vi "CLD 13 Flow Rates Exercise.vi"() -> ()   [LabVIEW 2009]
doc: "CLD 13 exercise"
panel:
  out "Error Out":errorcluster
  in  "Error In":errorcluster
  out "Flow Rate Meter":i8(knob) scale format="%_2f"
  in  "Stop Application":bool
  in  "Stop Flow":bool
  out "Elapsed Time":dbl
  out "Flow Rate":dbl
  in  "Flow Rate Change":i8(slide) min=-2 max=2 step=1
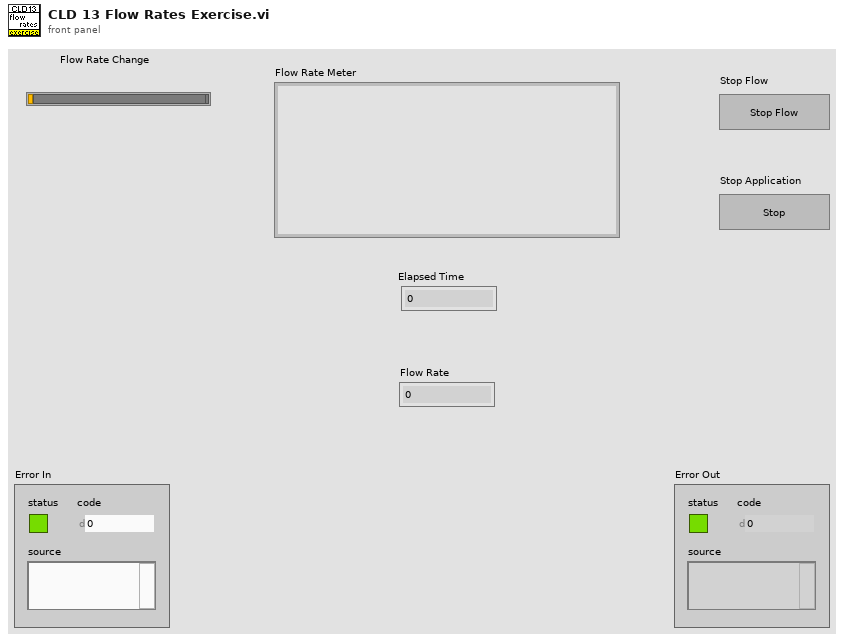
[diagram p1: front panel]
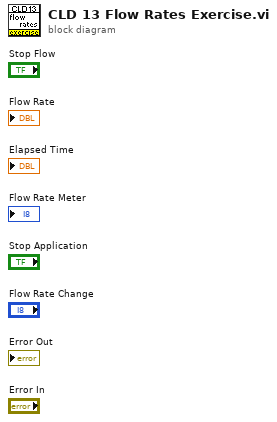
[diagram p0: block diagram]
diagram:
